vi "VMI_acquire_rewrite_v2.vi"(0 "IO settings":T1, 1 "Queue Array":T7[](array[typedef]), 3 "Peak Find Settings":T5, 9 "Collection Information":T6[](array[typedef]), 11 "error in":errorcluster, 12 "Ref Cluster 1":T4, 14 "Big_image Array":i16[][][](array[numeric])) -> (2 "Big_image Array Out":i16[][][](array[numeric]), 4 "Histogram":i32[][](array[numeric]), 6 "Peak Array":cluster{"X":sgl, "Y":sgl}[][](array[cluster]), 8 "Powers":dbl[][](array[numeric]), 10 "Power Err":dbl[][](array[numeric]), 13 "xaxis":i32[][](array[numeric]), 15 "error IO":errorcluster)   [LabVIEW 2020]
doc: "This VI collects the images, finds the number of counts in each image"
uses:
  Type defs/FileAcq_v1_Ctrl.ctl
  Type defs/Ref_cluster.ctl
  Type defs/IO_settings_ctrl.ctl
  <vilib>/vision/Image Controls.llb/IMAQ Image.ctl
  <vilib>/userdefined/High Color/IMAQdx.ctl
panel:
  out "XY Graph":cluster{"Y":dbl[], "Y":dbl[]}[](graph)
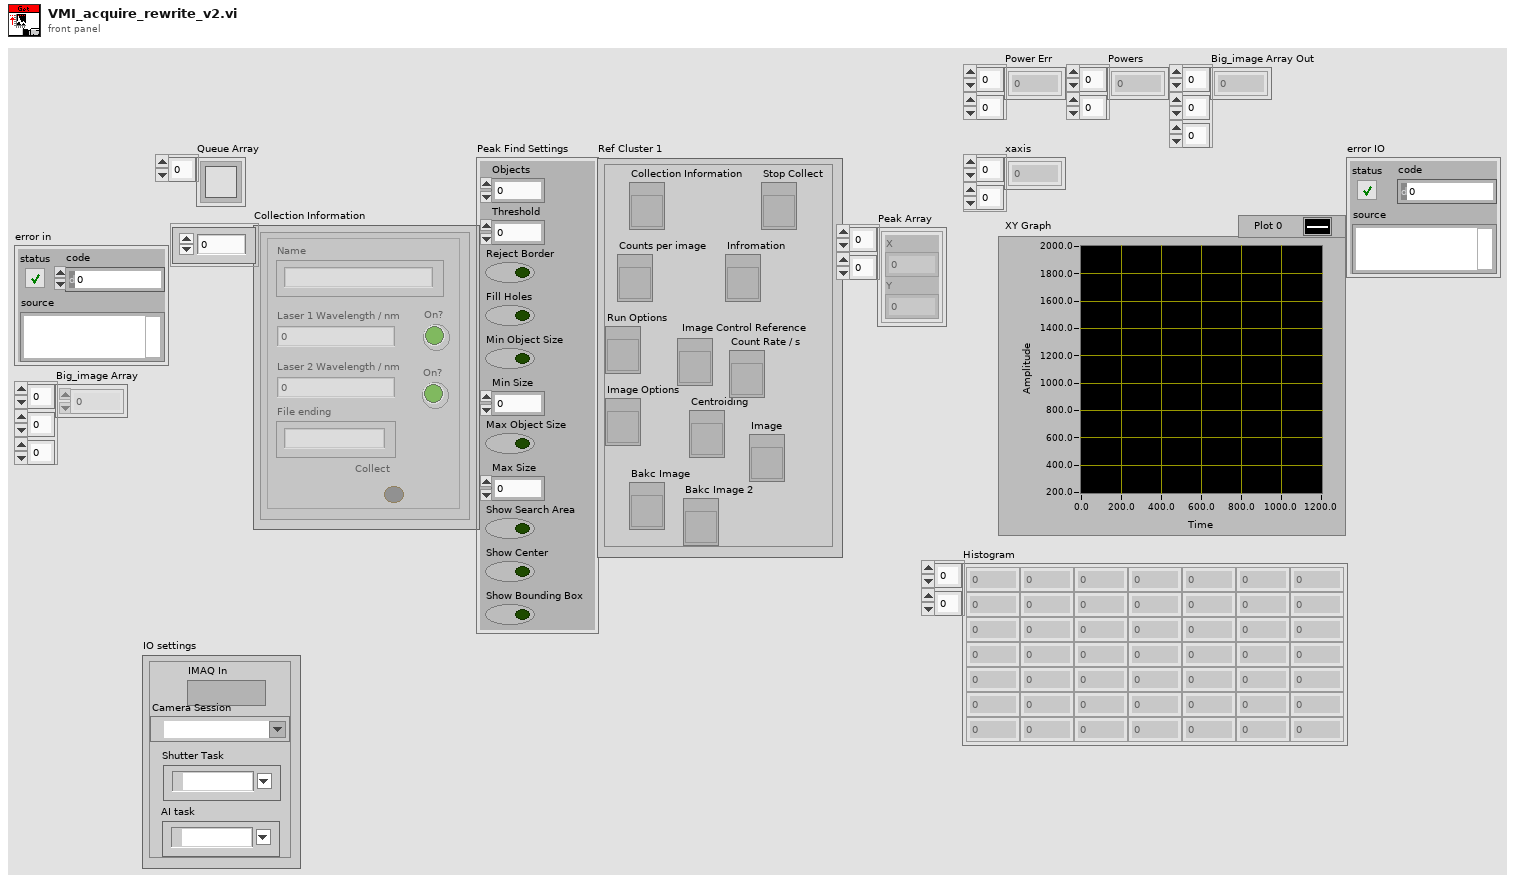
[diagram p1: front panel]
types:
  T1 = typedef "IO_settings_ctrl.ctl" = cluster{"IMAQ In":T2, "Camera Session":T3, "Shutter Task":refnum<k21>, "AI task":refnum<k21>}
  T2 = typedef "IMAQ Image.ctl" = refnum<image>
  T3 = typedef "IMAQdx.ctl" = refnum<k21>
  T4 = typedef "Ref_cluster.ctl" = cluster{"Stop Collect ":refnum<vi>, "Collection Information ":refnum<vi>, "Infromation":refnum<vi>, "Counts per image":refnum<vi>, " Image Control Reference ":refnum<vi>, "Run Options":refnum<vi>, "Image Options":refnum<vi>, "Centroiding":refnum<vi>, "Image":refnum<vi>, "Bakc Image":refnum<vi>, "Bakc Image 2":refnum<vi>, "Count Rate / s":refnum<vi>}
  T5 = cluster{"Objects":u16, "Threshold":i32, "Reject Border":bool, "Fill Holes":bool, "Min Object Size":bool, "Min Size":i32, "Max Object Size":bool, "Max Size":i32, "Show Search Area":bool, "Show Center":bool, "Show Bounding Box":bool}
  T6 = typedef "FileAcq_v1_Ctrl.ctl" = cluster{"Type":string, "LaserWave1":dbl, "Shutter1":bool, "LaserWave2":dbl, "Shutter2":bool, "FileEnd":string, "Collect":bool}
  T7 = typedef "Queue RefNum" = refnum<k1>
  T8 = typedef "Image Type" = u32
  T9 = cluster{"Total Time / ms":dbl, "Image Total Collection Time":dbl, "Image Loop time / ms":dbl, "Peak Total Find Time":dbl, "Peak Find Time / ms":dbl, "Camera Rate / Hz":dbl, "Total Number of Loops":dbl, "Current Loop Number":dbl, "Number of Image Loops":dbl, "Run Mode":dbl}
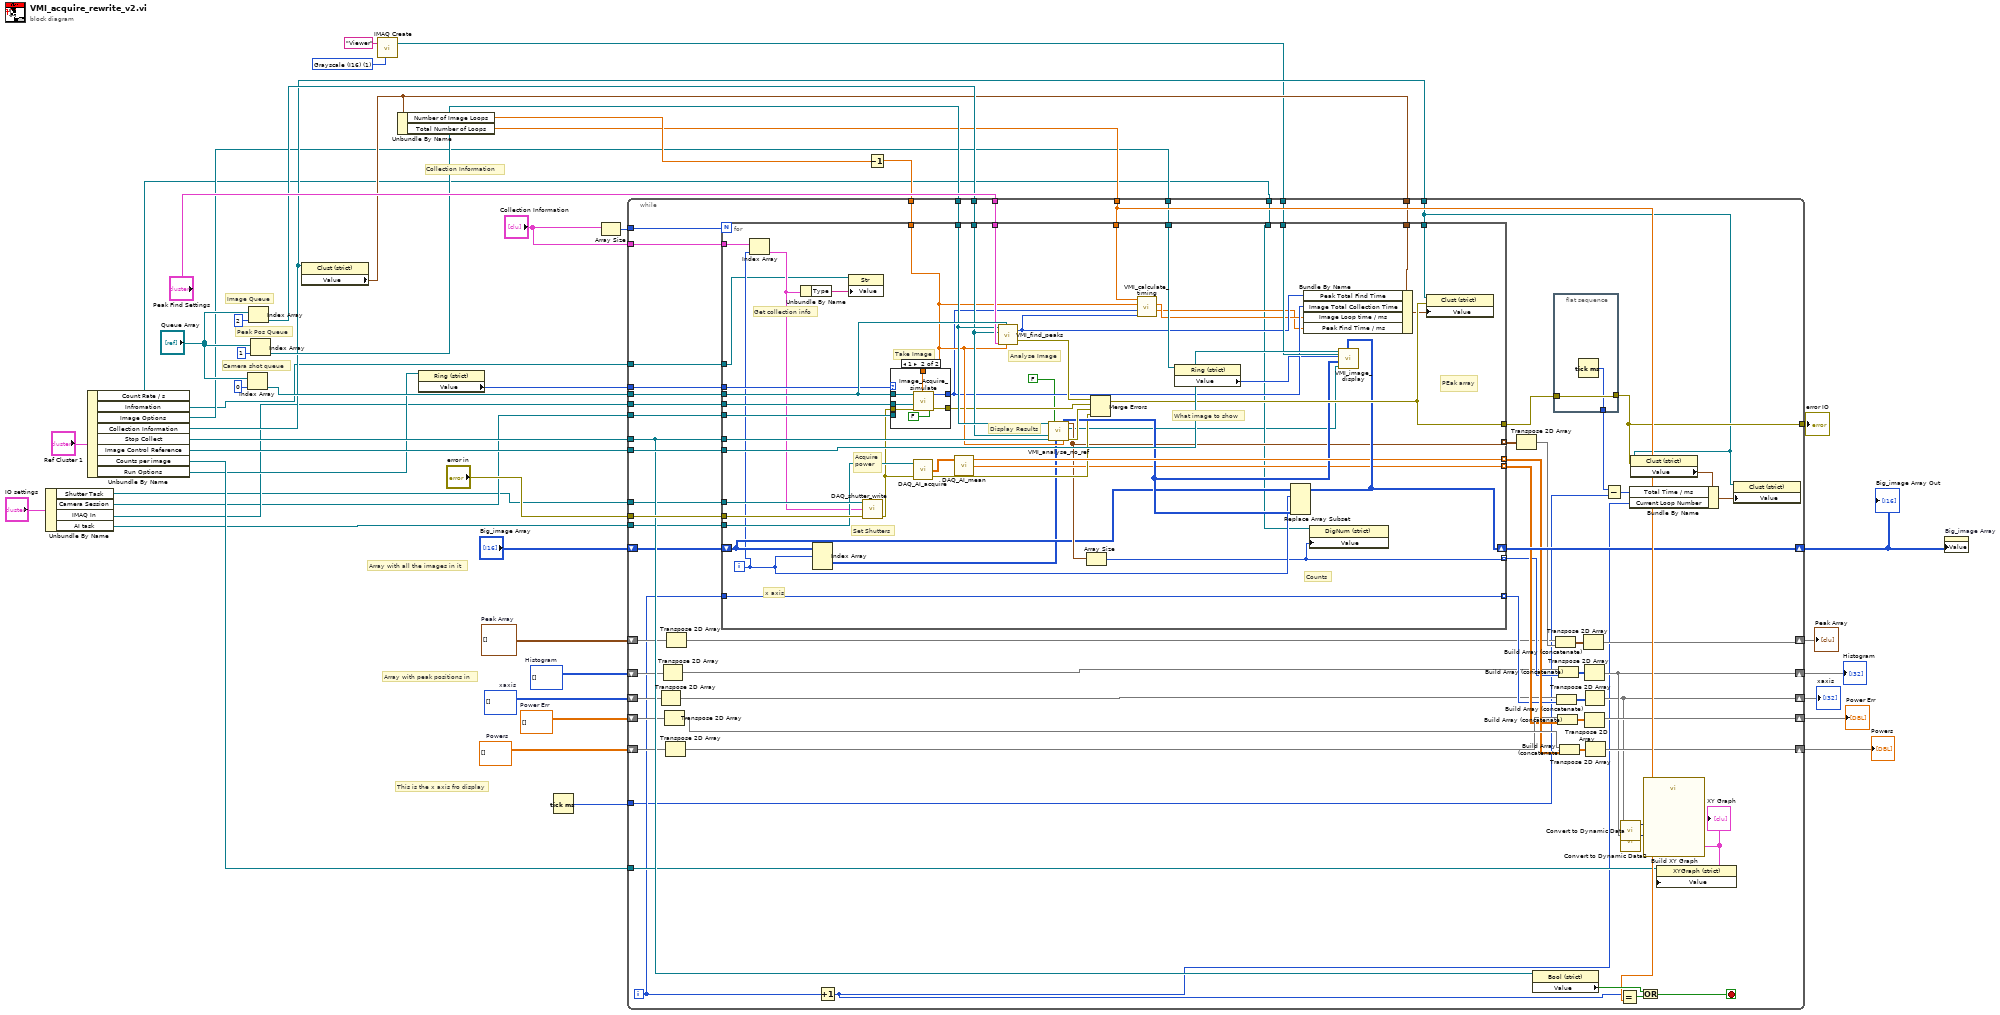
[diagram p0: block diagram]
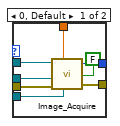
[diagram p2: hidden frame]
diagram:
  w6 = dbl[][] []  # Power Err
  w7 = dbl[][] []  # Powers
  w16 = T8 1 items=["Grayscale (U8)", "Grayscale (I16)", "Grayscale (SGL)", "Complex (CSG)", "RGB (U32)", "HSL (U32)", "RGB (U64)", "Grayscale (U16)"] ("Image Type")
  w8 = i32[][] []  # xaxis
  w26 = i32[][] []  # Histogram
  w28 = cluster{"X":sgl, "Y":sgl}[][] []  # Peak Array
  # "Array with all the images in it"
  # "Array with peak positions in"
  # "This is the x axis fro display"
  # "Collection Information"
  # "Image Queue"
  # "Peak Pos Queue"
  # "Camera shot queue"
  n1 = Unbundle By Name("IO settings") -> ("Shutter Task"=w10:refnum<k21>, "Camera Session"=w11:T3, "IMAQ In"=w12:T2, "AI task"=w9:refnum<k21>)
  n2 = Unbundle By Name("Ref Cluster 1") -> ("Count Rate / s"=w1:refnum<vi>, "Infromation"=w2:refnum<vi>, "Image Options"=w14:refnum<vi>, "Collection Information"=w30:refnum<vi>, "Stop Collect"=w36:refnum<vi>, "Image Control Reference"=w35:refnum<vi>, "Counts per image"=w27:refnum<vi>, "Run Options"=w19:refnum<vi>)
  n3 = Index Array(array="Queue Array", index=0) -> (element=w45:T7)
  n4 = Index Array(array="Queue Array", index=2) -> (element=w38:T7)
  n5 = Index Array(array="Queue Array", index=1) -> (element=w41:T7)
  n6 = property class="Clust (strict)"(reference=w30) -> ("Value"=w31:T9)  [unwired: 1 in, 2 out]
  n7 = call "IMAQ Create"("Image Name"="Viewer", "Image Type"=w16) -> ("New Image"=w15:T2)  [unwired: 3 in, 1 out]
  n8 = Unbundle By Name(w31) -> ("Number of Image Loops"=w34:dbl, "Total Number of Loops"=w32:dbl)
  n9 = property class="Ring (strict)"(reference=w19) -> ("Value"=w18:u16)  [unwired: 1 in, 2 out]
  n10 = Tick Count (ms)() -> (millisecond timer value=w3:u32)
  n11 = Array Size(array="Collection Information") -> (size(s)=w29:i32)
  n12 = Decrement(x=w34) -> (x-1=w33:dbl)
  n13 = while {
    tunnel: w12 -> [w113]
    tunnel: w11 -> [w112]
    tunnel: "error in" -> [w111]
    tunnel: w45 -> [w110]
    tunnel: "Collection Information" -> [w109]
    tunnel: "Peak Find Settings" -> [w108]
    tunnel: w41 -> [w107]
    tunnel: w38 -> [w106]
    tunnel: w36 -> [w103]
    tunnel: w35 -> [w105]
    tunnel: w33 -> [w104]
    tunnel: w32 -> [w100]
    tunnel: w31 -> [w59]
    tunnel: w30 -> [w51]
    tunnel: w29 -> [w95]
    tunnel: w27 -> [w67]
    shift-right: [w61] -> w20
    shift-left: w28 -> [w72]
    shift-right: [w69] -> w21
    shift-left: w26 -> [w77]
    shift-right: [w66] -> w25
    shift-left: w8 -> [w79]
    tunnel: [w52] -> w24
    shift-right: [w99] -> w22
    shift-left: "Big_image Array" -> [w98]
    tunnel: w18 -> [w97]
    tunnel: w15 -> [w94]
    tunnel: w14 -> [w93]
    tunnel: w10 -> [w92]
    tunnel: w9 -> [w91]
    shift-right: [w86] -> w4
    shift-left: w7 -> [w85]
    shift-right: [w81] -> w5
    shift-left: w6 -> [w90]
    tunnel: w3 -> [w55]
    tunnel: w2 -> [w49]
    tunnel: w1 -> [w48]
    i -> [w58]
    stop <- w96 stop-if-true
    n14 = Transpose 2D Array(2D array=w79) -> (transposed array=w78:i32[][])
    n15 = Transpose 2D Array(2D array=w77) -> (transposed array=w75:i32[][])
    n16 = Transpose 2D Array(2D array=w90) -> (transposed array=w89:dbl[][])
    n17 = Transpose 2D Array(2D array=w85) -> (transposed array=w84:dbl[][])
    n18 = Transpose 2D Array(2D array=w72) -> (transposed array=w63:cluster{"X":sgl, "Y":sgl}[][])
    n19 = for {
      N: w95 -> [_]
      tunnel: w113 -> [w163]
      tunnel: w112 -> [w162]
      tunnel: w111 -> [w161]
      tunnel: w110 -> [w160]
      tunnel: w109 -> [w123]
      tunnel: w108 -> [w159]
      tunnel: w107 -> [w158]
      tunnel: w106 -> [w157]
      tunnel: w103 -> [w156]
      tunnel: w105 -> [w155]
      tunnel: w104 -> [w154]
      tunnel: w100 -> [w153]
      tunnel: w58 -> [w127]
      tunnel: w59 -> [w152]
      tunnel: w51 -> [w151]
      tunnel: [w150] -> w53
      shift-right: [w149] -> w99
      shift-left: w98 -> [w125]
      tunnel: w97 -> [w148]
      tunnel: w94 -> [w147]
      tunnel: w93 -> [w146]
      tunnel: w92 -> [w145]
      tunnel: w91 -> [w144]
      tunnel: [w143] -> w88 mode=indexing
      tunnel: [w128] -> w83 mode=indexing
      tunnel: [w127] -> w80 mode=indexing
      tunnel: [w117] -> w76 mode=indexing
      tunnel: [w126] -> w73 mode=indexing
      tunnel: w49 -> [w120]
      tunnel: w48 -> [w118]
      i -> [w121]
      # "Acquire\npower"
      # "Set Shutters"
      # "What image to show"
      # "x axis"
      # "Counts"
      # "PEak array"
      # "Display Results"
      # "Analyse Image"
      # "Take Image"
      # "Get collection info"
      # "This loop collects for each required image"
      n20 = Index Array(array=w123, index=w121) -> (element=w122:T6)
      n21 = Unbundle By Name(w122) -> ("Type"=w119:string)
      n22 = Index Array(array=w125, index (dim 0)=w121) -> (element=w124:i16[][])  [unwired: 2 in]
      n23 = property class="Str"(reference=w120, "Value"=w119) -> ()  [unwired: 1 in, 2 out]
      n24 = call "DAQ_shutter_write.vi"("Error In"=w161, "Collection Settings"=w122, "DAQmx Task Name"=w145) -> ("Error Out"=w131:errorcluster)  [unwired: 2 in]
      n25 = case shown="1" w148 {
        tunnel: w163 -> [w170 w172]
        tunnel: w162 -> [w169 _]
        tunnel: w131 -> [w168 w178]
        tunnel: w160 -> [w167 w174]
        tunnel: [w166 w177] -> w141
        tunnel: w154 -> [w165 w175]
        tunnel: [w164 w176] -> w138
        frame 0, Default {
          n26 = call "Image_Acquire.vi"("Queue Ref in"=w167, "Acquire Time"=w165, "Image Out"=w170, "Session In"=w169, "error in (no error)"=w168, "Test Timing"=FALSE) -> ("Loop Time Out"=w164:i64, "error out"=w166:errorcluster)  [unwired: 1 in]
        }
        frame 1 {
          n27 = call "Image_Acquire_simulate.vi"("Queue Ref in"=w174, "Acquire Time"=w175, "Image Out"=w172, "error in (no error)"=w178, "Test Timing"=FALSE) -> ("Loop Time Out"=w176:i64, "error out"=w177:errorcluster)  [unwired: 2 in]
        }
      }
      n28 = call "DAQ_AI_acquire.vi"("Error In"=w131, "DAQmx Task Name"=w144) -> ("Error Out"=w129:errorcluster, "data"=w130:dbl[][])  [unwired: 1 in, 1 out]
      n29 = call "DAQ_AI_mean.vi"("data"=w130) -> ("Std"=w128:dbl[], "Mean"=w143:dbl[])  [unwired: 3 in]
      n30 = call "VMI_find_peaks.vi"("Acquire Time"=w154, "Acquire Queue In"=w160, "Peak Find Settings"=w159, "Image Queue in"=w157, "Peak Position Queue in"=w158) -> ("error out"=w142:errorcluster, "x-y"=w139:u32)  [unwired: 1 in]
      n31 = call "VMI_analyse_no_ref.vi"("Peak Position Queue in"=w158, "Test Timing"=FALSE, "Image in"=w157, "Stop Button Ref"=w156, "Image_array"=w124, "Acquire Time"=w154) -> ("Image_array out"=w133:i32[][], "Peaks Position Out"=w126:cluster{"X":sgl, "Y":sgl}[], "Current Image"=w116:T2, "error out"=w140:errorcluster)  [unwired: 5 in, 1 out]
      n32 = Array Size(array=w126) -> (size(s)=w117:i32)
      n33 = Merge Errors(w142, w141, w140, w129) -> (w150:errorcluster)
      n34 = call "VMI_calculate_timing.vi"("Peakfind total time"=w139, "Camera_Total_loop time"=w138, "Number of image loops"=w154, "Total loop Number"=w153) -> ("AveragePeak find time"=w136:dbl, "Average Image Loop time"=w137:dbl)  [unwired: 1 in, 1 out]
      n35 = property class="Ring (strict)"(reference=w146) -> ("Value"=w132:u16)  [unwired: 1 in, 2 out]
      n36 = Replace Array Subset(array=w125, new element=w133, index (dim 0)=w121) -> (w149:i16[][][])  [unwired: 2 in]
      n37 = Bundle By Name(cluster=w152, "Peak Total Find Time"=w139, "Image Total Collection Time"=w138, "Image Loop time / ms"=w137, "Peak Find Time / ms"=w136) -> (w135:T9)
      n38 = property class="DigNum (strict)"(reference=w118, "Value"=w117) -> ()  [unwired: 1 in, 2 out]
      n39 = call "VMI_image_display.vi"("Image_control"=w155, "Image to show"=w132, 2:"Current Image"=w133, 3:"Current Image"=w116, "Big_image Array"=w149, "Canvas"=w147) -> ()  [unwired: 4 in, 1 out]
      n40 = property class="Clust (strict)"(reference=w151, error in=w150, "Value"=w135) -> ()  [unwired: 2 out]
    }
    n41 = Increment(x=w58) -> (x+1=w57:i32)
    n42 = Transpose 2D Array(2D array=w73) -> (transposed array=w64:cluster{"X":sgl, "Y":sgl}[][])
    n43 = property on="Property Node" class="Bool (strict)"(reference=w103) -> ("Value"=w102:bool)  [unwired: 1 in, 2 out]
    n44 = flat-sequence {
      tunnel: w53 -> [w115]
      tunnel: [w115] -> w52
      tunnel: [w114] -> w50
      frame #0 {
        n45 = Tick Count (ms)() -> (millisecond timer value=w114:u32)
      }
    }
    n46 = Build Array (concatenate)(w63, w64) -> (w62:cluster{"X":sgl, "Y":sgl}[][])
    n47 = Build Array (concatenate)(w78, w80) -> (w70:i32[][])
    n48 = Build Array (concatenate)(w84, w83) -> (w82:dbl[][])
    n49 = Build Array (concatenate)(w75, w76) -> (w74:i32[][])
    n50 = Build Array (concatenate)(w89, w88) -> (w87:dbl[][])
    n51 = Transpose 2D Array(2D array=w62) -> (transposed array=w61:cluster{"X":sgl, "Y":sgl}[][])
    n52 = Transpose 2D Array(2D array=w74) -> (transposed array=w69:i32[][])
    n53 = Transpose 2D Array(2D array=w82) -> (transposed array=w81:dbl[][])
    n54 = Transpose 2D Array(2D array=w70) -> (transposed array=w66:i32[][])
    n55 = Transpose 2D Array(2D array=w87) -> (transposed array=w86:dbl[][])
    n56 = Subtract(x=w50, y=w55) -> (x-y=w56:u32)
    n57 = Equal?(x=w57, y=w100) -> (x = y?=w101:bool)
    n58 = call "Convert to Dynamic Data2"("2D Array"=w69) -> ("Dynamic Data Type"=w68:dynamicdata)  [unwired: 3 in]
    n59 = call "Convert to Dynamic Data"("2D Array"=w66) -> ("Dynamic Data Type"=w65:dynamicdata)  [unwired: 3 in]
    n60 = property class="Clust (strict)"(reference=w51, error in=w52) -> ("Value"=w54:T9)  [unwired: 2 out]
    n61 = Bundle By Name(cluster=w54, "Total Time / ms"=w56, "Current Loop Number"=w57) -> (w60:T9)
    n62 = Or(x=w102, y=w101) -> (x .or. y?=w96:bool)
    n63 = call "Build XY Graph"("Y Input"=w68, "X Input"=w65) -> ("XY Graph"=w71:cluster{"X":dbl[], "Y":dbl[]}[])  [unwired: 8 in, 1 out]
    "XY Graph" <- w71
    n64 = property on="Property Node" class="XYGraph (strict)"(reference=w67, "Value"=w71) -> ()  [unwired: 1 in, 2 out]
    n65 = property class="Clust (strict)"(reference=w51, "Value"=w60) -> ()  [unwired: 1 in, 2 out]
  }
  "Histogram" <- w21
  "Peak Array" <- w20
  "xaxis" <- w25
  "error IO" <- w24
  "Power Err" <- w5
  "Powers" <- w4
  "Big_image Array Out" <- w22
  n66 = property on="Big_image Array" class="Arr (strict)"("Value"=w22) -> ()  [unwired: 2 in, 2 out]
